vi "MCL Single Write N.vi"(9 "handle":i32, 10 "axis":u32, 11 "position":dbl) -> (3 "function return":i32)   [LabVIEW 2017, in "Madlib.lvlib"]
doc: "MADLIB_API int MCL_SingleWriteN(double position, unsigned int axis, int handle);"
uses:
  Madlib.lvlib
  Madlib.dll
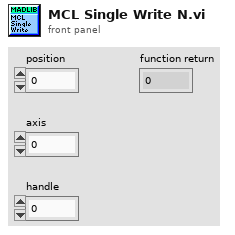
[diagram p1: front panel]
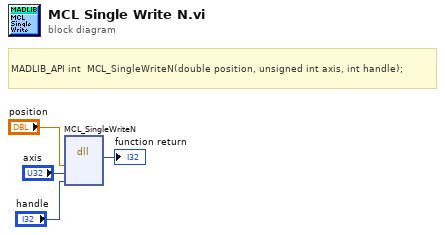
[diagram p0: block diagram]
diagram:
  # "MADLIB_API\tint\t\tMCL_SingleWriteN(double position, unsigned int axis, int handle);"
  n1 = dll-call lib="C:/Users/francesco/dev/pump-probe/Piezo/lvlib/Madlib.*" fn="MCL_SingleWriteN"("position"="position", "axis"="axis", "handle"="handle") -> (→"function return":i32)  [unwired: 6 in, 2 out]
